vi "disable messages.vi"(11 "message to check":string) -> (3 "message out":string)   [LabVIEW 2013, in "configuration library.lvlib"]
uses:
  configuration library.lvlib
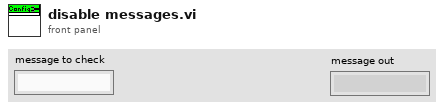
[diagram p1: front panel]
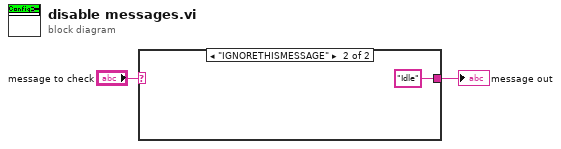
[diagram p0: block diagram]
diagram:
  n1 = case shown="\"IGNORETHISMESSAGE\"" "message to check" {
    selector: "message to check" -> [w3 _]
    tunnel: [w3 "Idle"] -> w1
    frame Default {
    }
    frame "IGNORETHISMESSAGE" {
    }
  }
  "message out" <- w1
